vi "Handle Message.vi"(8 "error in (no error)":errorcluster, 9 "Message Completion Handler":refnum<class "Message Completion Handler.lvclass">, 10 "Message":string, 11 "Plugin In":refnum<class "Sift TDMS Uploader.lvclass">) -> (0 "error out":errorcluster, 1 "Synchronously Complete Message?":bool=TRUE, 2 "Message Response":string, 3 "Plugin out":refnum<class "Sift TDMS Uploader.lvclass">)   [LabVIEW 2024, in "Sift TDMS Uploader.lvlib" / "Sift TDMS Uploader.lvclass"]
uses:
  Sift TDMS Uploader.lvclass
  <vilib>/FlexLogger/SDK/PluginSDK.lvlibp/PEFClasses/SDK/Message Completion Handler/Message Completion Handler.lvclass
  Sift TDMS Uploader.lvclass/Sift TDMS Uploader.ctl
  SubVIs/Log Event Types.ctl
  Globals.vi
  <vilib>/FlexLogger/SDK/PluginSDK.lvlibp/PEFClasses/SDK/Processing Element/Read System Interface.vi
  <vilib>/FlexLogger/SDK/PluginSDK.lvlibp/PEFClasses/SDK/Processing Element/Read Alias.vi
  <vilib>/FlexLogger/SDK/PluginSDK.lvlibp/PEFClasses/SDK/System Interface/System Interface.lvclass
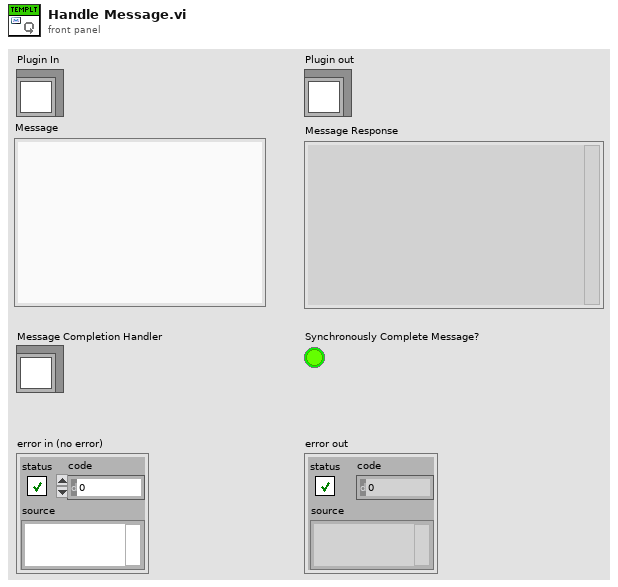
[diagram p1: front panel]
types:
  T1 = typedef "Sift TDMS Uploader.lvlib/Sift TDMS Uploader.lvclass/Log Event Types.ctl" = enum16{"INFO", "WARN", "ERROR"}
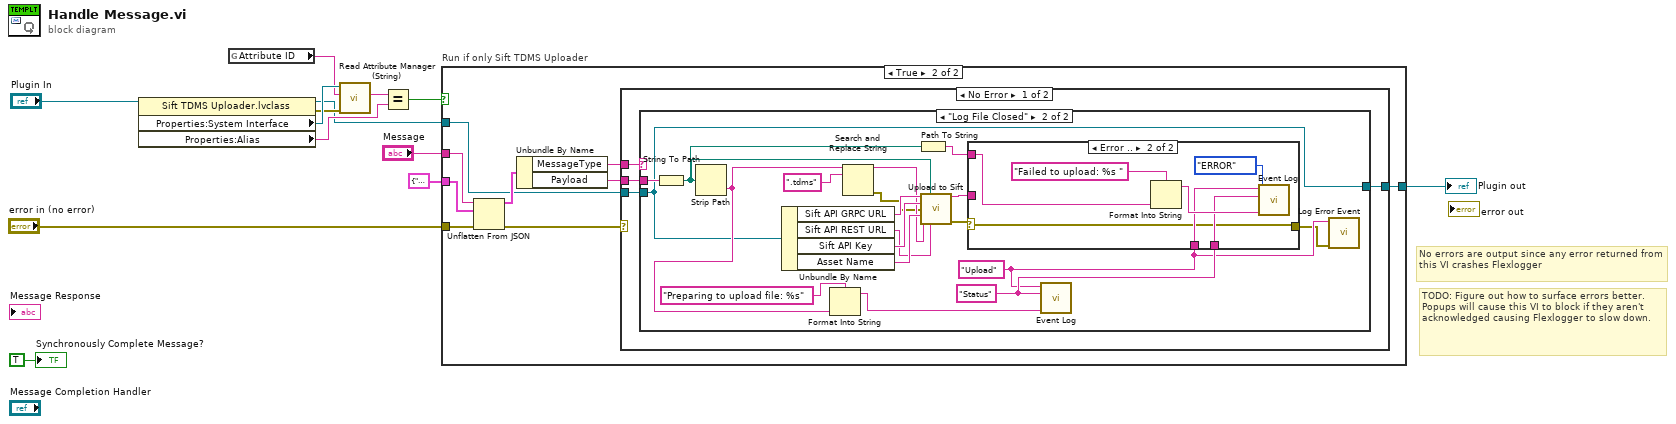
[diagram p0: block diagram]
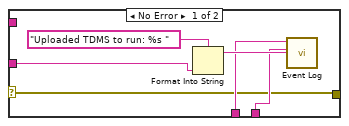
[diagram p4: hidden frame]
diagram:
  # "TODO: Figure out how to surface errors better. Popups will cause this VI to block if they aren't acknowledged causing Flexlogger to slow down."
  # "No errors are output since any error returned from this VI crashes Flexlogger"
  n1 = property class="Sift TDMS Uploader.lvclass"(reference="Plugin In") -> (reference out=w1:refnum<class "Sift TDMS Uploader.lvclass">, error out=w11:errorcluster, "Properties:System Interface"=w12:refnum<class "System Interface.lvclass">, "Properties:Alias"=w3:string)  [unwired: 1 in]
  n2 = global read "Globals.vi" "Attribute ID"() -> (w10:string)
  n3 = call-dynamic "Read Attribute Manager (String).vi"("error in (no error)"=w11, "Attribute ID"=w10, "System Interface in"=w12) -> ("Attrib Val"=w4:string)  [unwired: 5 in, 3 out]
  n4 = Equal?(x=w4, y=w3) -> (x = y?=w9:bool)
  n5 = case "Run if only Sift TDMS Uploader" shown="True" w9 {
    tunnel: w1 -> [w14 w19]
    tunnel: "Message" -> [_ w18]
    tunnel: cluster{"Payload":string, "MessageType":string} {"Payload"="", "MessageType"=""} -> [_ w17]
    tunnel: "error in (no error)" -> [_ w16]
    tunnel: [w14 w15] -> w5
    frame False {
    }
    frame True {
      n6 = Unflatten From JSON(JSON string=w18, type and defaults=w17, error in (no error)=w16) -> (value=w20:cluster{"Payload":string, "MessageType":string}, error out=w21:errorcluster)  [unwired: 4 in]
      n7 = Unbundle By Name(w20) -> ("MessageType"=w22:string, "Payload"=w23:string)
      n8 = case shown="No Error" w21 {
        tunnel: w22 -> [w27 _]
        tunnel: w23 -> [w25 _]
        tunnel: w19 -> [w26 w61]
        tunnel: [w24 w61] -> w15
        frame No Error {
          n9 = case shown="\"Log File Closed\"" w27 {
            tunnel: w25 -> [_ w47]
            tunnel: w26 -> [w28 w35]
            tunnel: [w28 w35] -> w24
            frame Default {
            }
            frame "Log File Closed" {
              w34 = "Status"
              w31 = "Upload"
              n10 = String To Path(string=w47) -> (path=w33:path)
              n11 = Strip Path(path=w33) -> (name=w37:string)  [unwired: 1 out]
              n12 = Unbundle By Name(w35) -> ("Sift API GRPC URL"=w46:string, "Sift API REST URL"=w43:string, "Sift API Key"=w45:string, "Asset Name"=w44:string)
              n13 = Format Into String(format string="Preparing to upload file: %s", w37) -> (resulting string=w36:string)  [unwired: 2 in, 1 out]
              n14 = Search and Replace String(input string=w37, search string=".tdms") -> (result string=w40:string, error out=w29:errorcluster)  [unwired: 6 in, 2 out]
              n15 = Path To String(path=w33) -> (string=w32:string)
              n16 = call "Upload to Sift.vi"("API GRPC URL"=w46, "Absolute Filepath"=w33, "API Key"=w45, "error in (no error)"=w29, "Asset Name"=w44, "Run Name"=w40, "API REST URL"=w43) -> ("Run URL"=w42:string, "Error"=w41:errorcluster)  [unwired: 7 in]
              n17 = case shown="Error .." w41 {
                selector: w41 -> [w48 w55]
                tunnel: w42 -> [w52 _]
                tunnel: w31 -> [w50 w56]
                tunnel: w34 -> [w49 w57]
                tunnel: w32 -> [_ w54]
                tunnel: [w48 w55] -> w30
                frame No Error {
                  n18 = Format Into String(format string="Uploaded TDMS to run: %s ", w52) -> (resulting string=w51:string)  [unwired: 2 in, 1 out]
                  n19 = call "Event Log.vi"("Message"=w51, "Event Type"=w49, "Location"=w50) -> ()  [unwired: 9 in]
                }
                frame Error {
                  n20 = Format Into String(format string="Failed to upload: %s ", w54) -> (resulting string=w59:string)  [unwired: 2 in, 1 out]
                  n21 = call "Event Log.vi"("Message"=w59, "Log Event Type"=Log_Event_Types."ERROR" ("Log Event Types"), "Event Type"=w57, "Location"=w56) -> ()  [unwired: 8 in]
                }
              }
              n22 = call "Event Log.vi"("Message"=w36, "Event Type"=w34, "Location"=w31) -> ()  [unwired: 9 in]
              n23 = call "Log Error Event.vi"("error in (no error)"=w30, "Location"=w31) -> ()  [unwired: 10 in]
            }
          }
        }
        frame Error {
        }
      }
    }
  }
  "Plugin out" <- w5
  "Synchronously Complete Message?" <- TRUE ("Synchronously Complete Message?")
